vi "Base64_EncodeAnything.vi"(8 "error in (no error)":errorcluster, 11 "Variant":variant) -> (0 "error out":errorcluster, 2 "Encoded Payload":string, 3 "Variant dup":variant)   [LabVIEW 2017, in "Serializer.Base64.lvclass"]
doc: "20250509 - Added default Base64 charset"
uses:
  Serializer.Base64.lvclass
  C:/Program Files (x86)/National Instruments/LabVIEW 2024/vi.lib/LabVIEW Open Source Project/OpenSerializer/Serializer/Serializer.lvclass
  Serializer.Base64.lvclass/Serializer.Base64.ctl
  <vilib>/LabVIEW Open Source Project/OpenSerializer/Serializer/Serializer.lvclass
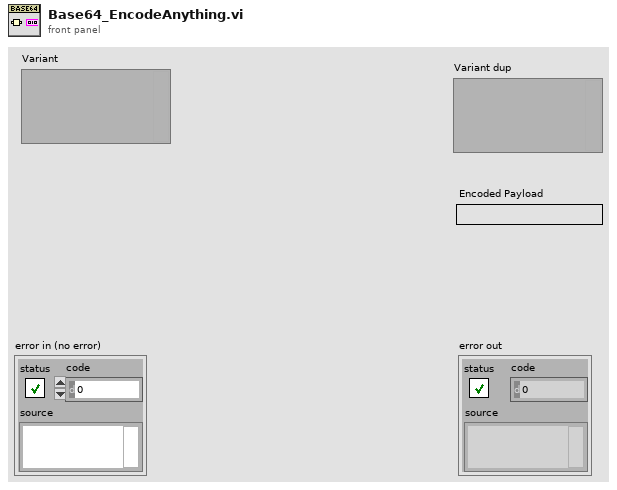
[diagram p1: front panel]
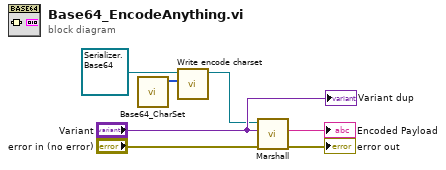
[diagram p0: block diagram]
diagram:
  n1 = call "Base64_CharSet.vi"() -> ("Base64 charset"=w3:u8[])  [unwired: 11 in]
  n2 = call "Write encode charset.vi"("encode charset"=w3, "Serializer.Base64 in"=refnum<class "Serializer.Base64.lvclass"> refnum) -> ("Serializer.Base64 out"=w1:refnum<class "Serializer.Base64.lvclass">)  [unwired: 8 in, 1 out]
  n3 = call <vilib>:"Marshall.vi"("error in (no error)"="error in (no error)", "Variant"="Variant", "Serializer in"=w1) -> ("error out"=→"error out":errorcluster, "String"=→"Encoded Payload":string)  [unwired: 6 in, 1 out]
  "Variant dup" <- "Variant"
